vi "runTestScenario.vi"(8 "error in (no error)":errorcluster, 11 "RS232-RXD High Test in":refnum<class "RS232-RXD High Test.lvclass">) -> (0 "error out":errorcluster, 2 "TestExecution":T1, 3 "RS232-RXD High Test out":refnum<class "RS232-RXD High Test.lvclass">)   [LabVIEW 2015, in "RS232-RXD High Test.lvclass"]
uses:
  RS232-RXD High Test.lvclass
  Typedefs/TestExecution.ctl
  RS232-RXD High Test.lvclass/RS232-RXD High Test.ctl
  <userlib>/Common/ilc/Typedefs/DigitalOutputValues.ctl
  Typedefs/WriteLogMessageInput.ctl
  Typedefs/TestScenarioTypes.ctl
  Typedefs/PassFailTest.ctl
  Model/TestLog/ITestLog/ITestLog.lvclass
  Typedefs/ILCBTTypedefs.lvlib
  <userlib>/Common/ilc/ILC/ILC.lvclass
  <userlib>/Common/ilc/Typedefs/ILCTypedefs.lvlib
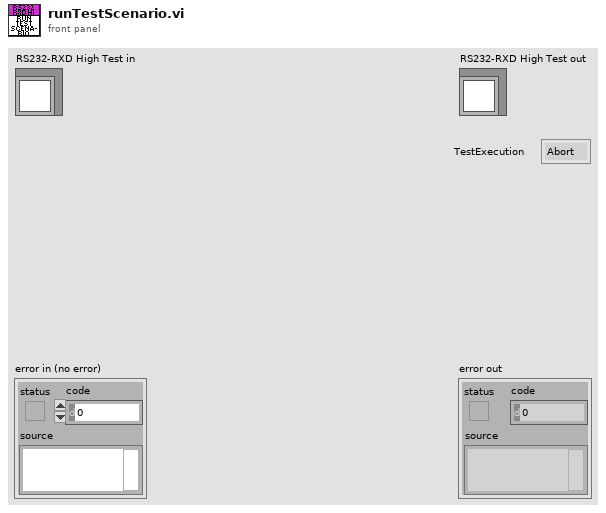
[diagram p1: front panel]
types:
  T1 = typedef "ILCBTTypedefs.lvlib/TestExecution.ctl" = enum16{"Abort", "Continue"}
  T2 = typedef "ILCBTTypedefs.lvlib/Digital Signal Level.ctl" = enum16{"Low", "High"}
  T3 = typedef "ILCBTTypedefs.lvlib/MUX Settings.ctl" = cluster{"MUX_AO":T2, "MUX_A1":T2, "MUX_A0 DAQ Channel to Write":refnum<k21>, "MUX_A1 DAQ Channel to Write":refnum<k21>}
  T4 = typedef "ILCBTTypedefs.lvlib/WriteLogMessageInput.ctl" = cluster{"Test Scenario":T5, "Description":string, "Actual Value":string, "Data File":string, "Result":T6}
  T5 = typedef "ILCBTTypedefs.lvlib/TestScenarioTypes.ctl" = enum16{"+3.3VA Supply Test", "+3.3VD Supply Test", "+5VA Supply Test", "+5VD Supply Test", "Unique ID Test", "TEDS Status Test", "LIMSW1_TTL Low Test", "LIMSW1_TTL High Test", "LIMSW2_TTL Low Test", "LIMSW2_TTL High Test", "Tachometer Test", "SSR_TTL Low Test", "SSR_TTL High Test", "SM_CW Low Test", "SM_CW High Test", "SM_CCW Low Test", "SM_CCW High Test", "SM_GPI Low Test", "SM_GPI High Test", "CW Motion Without Limit Test", "CW Motion With Limit Test", "CW Motion With Limit Interruption Test", "CW Motion on CCW Limit Test", "CCW Motion Without Limit Test", "CCW Motion With Limit Test", "CCW Motion With Limit Interruption Test", "CCW Motion on CW Limit Test", "RS232-TXD Low Test", "RS232-TXD High Test", "RS232-RTS Low Test", "RS232-RTS High Test", "RS232-RXD Low Test", "RS232-RXD High Test", "RS232-CTS Low Test", "RS232-CTS High Test", "Out_SS Low Test", "Out_SS High Test", "Out_SDI Low Test", "Out_SDI High Test", "Out_SCLK Low Test", "Out_SCLK High Test", "Reset Low Test", "Reset High Test", "1 Channel ADC Test", "3 Channel ADC Test", "5 Channel ADC Test", "Vref Test", "ROT Test", "DAC1 Test", "DAC2 Test", "DAC3 Test", "DAC4 Test", "BIAS Test", "EXC1 Test", "EXC2 Test", "EXC3 Test", "EXC4 Test"}
  T6 = typedef "ILCBTTypedefs.lvlib/PassFailTest.ctl" = enum16{"Fail", "Pass", "NA"}
  T7 = typedef "ILCCommon.lvlib/ILCTypedefs.lvlib/DigitalOutputValues.ctl" = cluster{"All Off":bool, "SM_CW":bool, "SM_CCW":bool, "UART2_TXD":bool, "UART2_RTS":bool, "UART2_RXD":bool, "UART2_CTS":bool, "OUT_SDO":bool, "OUT_SDI":bool, "OUT_SCK":bool, "MB_SS":bool, "MB_RESET":bool, "SSR_OUT":bool}
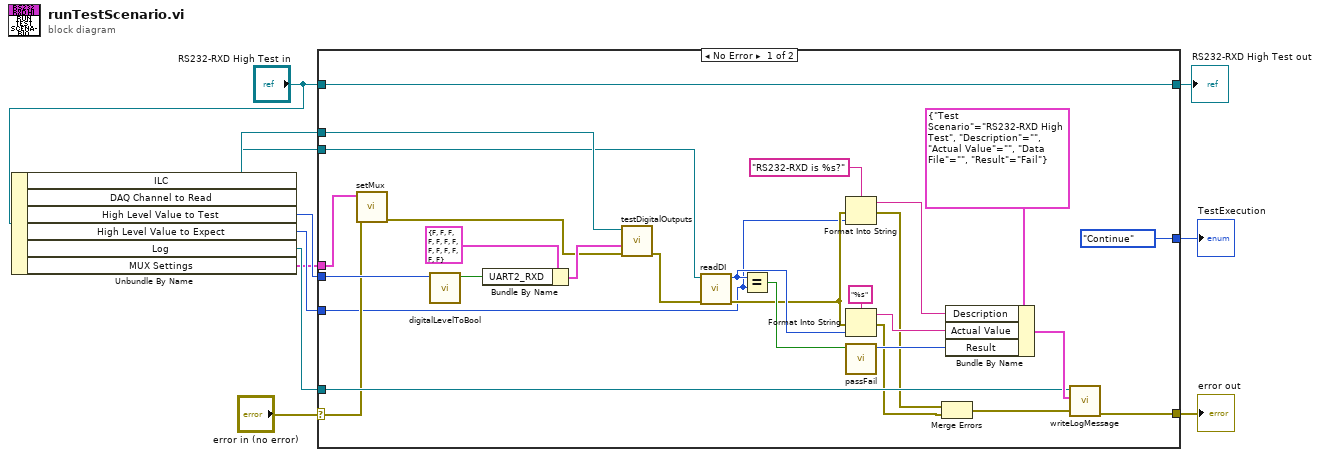
[diagram p0: block diagram]
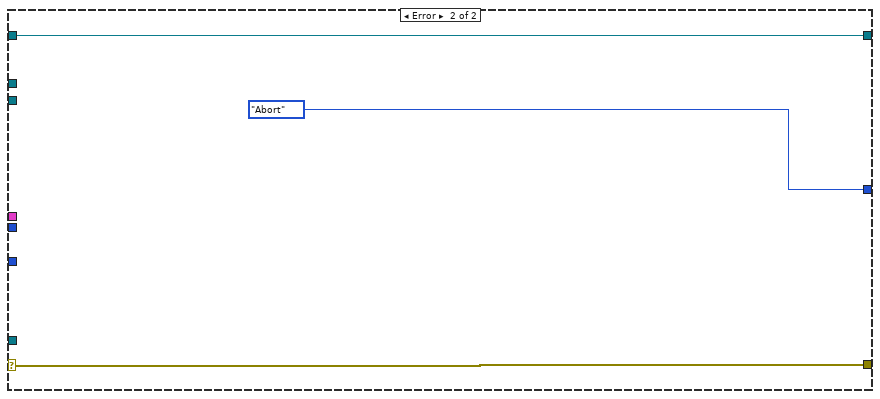
[diagram p2: hidden frame]
diagram:
  n1 = Unbundle By Name("RS232-RXD High Test in") -> ("ILC"=w5:refnum<class "ILC.lvclass">, "DAQ Channel to Read"=w4:refnum<k21>, "High Level Value to Test"=w6:T2, "High Level Value to Expect"=w3:T2, "Log"=w2:refnum<class "ITestLog.lvclass">, "MUX Settings"=w1:T3)
  n2 = case shown="No Error" "error in (no error)" {
    selector: "error in (no error)" -> [w19 w41]
    tunnel: [w23 w41] -> w10
    tunnel: [w37 w42] -> w9
    tunnel: "RS232-RXD High Test in" -> [w37 w42]
    tunnel: [TestExecution."Continue" ("TestExecution") TestExecution."Abort" ("TestExecution")] -> w8
    tunnel: w6 -> [w34 _]
    tunnel: w5 -> [w33 _]
    tunnel: w4 -> [w31 _]
    tunnel: w3 -> [w12 _]
    tunnel: w2 -> [w22 _]
    tunnel: w1 -> [w21 _]
    frame No Error {
      n3 = call "setMux.vi"("error in (no error)"=w19, "MUX Settings"=w21) -> ("error out"=w20:errorcluster)  [unwired: 9 in]
      n4 = call "digitalLevelToBool.vi"("Digital Signal Level"=w34) -> ("Bool?"=w35:bool)  [unwired: 10 in]
      n5 = Bundle By Name(cluster=T7 {"All Off"=FALSE, "SM_CW"=FALSE, "SM_CCW"=FALSE, "UART2_TXD"=FALSE, "UART2_RTS"=FALSE, "UART2_RXD"=FALSE, "UART2_CTS"=FALSE, "OUT_SDO"=FALSE, "OUT_SDI"=FALSE, "OUT_SCK"=FALSE, "MB_SS"=FALSE, "MB_RESET"=FALSE, "SSR_OUT"=FALSE} ("Digital Output Values"), "UART2_RXD"=w35) -> (w32:T7)
      n6 = call <userlib>:"testDigitalOutputs.vi"("error in (no error)"=w20, "Digital Output Values"=w32, "ILC in"=w33) -> ("error out"=w38:errorcluster)  [unwired: 7 in, 1 out]
      n7 = call "readDI.vi"("error in (no error)"=w38, "DAQ Channel To Read"=w31) -> ("error out"=w14:errorcluster, "Digital Signal Level"=w27:T2)  [unwired: 8 in]
      n8 = Equal?(x=w27, y=w12) -> (x = y?=w28:bool)
      n9 = Format Into String(format string="RS232-RXD is %s?", error in=w14, w12) -> (resulting string=w18:string, error out=w15:errorcluster)  [unwired: 1 in]
      n10 = Format Into String(format string="%s", error in=w14, w27) -> (resulting string=w25:string, error out=w17:errorcluster)  [unwired: 1 in]
      n11 = call "passFail.vi"("Boolean"=w28) -> ("Result"=w29:T6)  [unwired: 10 in]
      n12 = Merge Errors(w15, w17) -> (w16:errorcluster)
      n13 = Bundle By Name(cluster=T4 {"Test Scenario"=enum."RS232-RXD High Test", "Description"="", "Actual Value"="", "Data File"="", "Result"=enum."Fail"} ("WriteLogMessageInput"), "Description"=w18, "Actual Value"=w25, "Result"=w29) -> (w24:T4)
      n14 = call-dynamic "writeLogMessage.vi"("error in (no error)"=w16, "WriteLogMessageInput"=w24, "ITestLog in"=w22) -> ("error out"=w23:errorcluster)  [unwired: 7 in, 1 out]
    }
    frame Error {
    }
  }
  "error out" <- w10
  "RS232-RXD High Test out" <- w9
  "TestExecution" <- w8
